vi "get.vi"(7 "save_to_file":path, 8 "error in (no error)":errorcluster, 10 "url":string, 11 "Client in":refnum<class "Client.lvclass">) -> (0 "error out":errorcluster, 2 "string_value":string, 3 "Client out":refnum<class "Client.lvclass">)   [LabVIEW 2020, in "reqwest.lvlib" / "Client.lvclass"]
uses:
  Client.lvclass
  Client.lvclass/Client.ctl
  lv_reqwest_64.dll
  reqwest.lvlib
  <userlib>/_OpenG.lib/file/file.llb/openg_file.lvlib
  <userlib>/_OpenG.lib/file/file.llb/Valid Path - Traditional__ogtk.vi
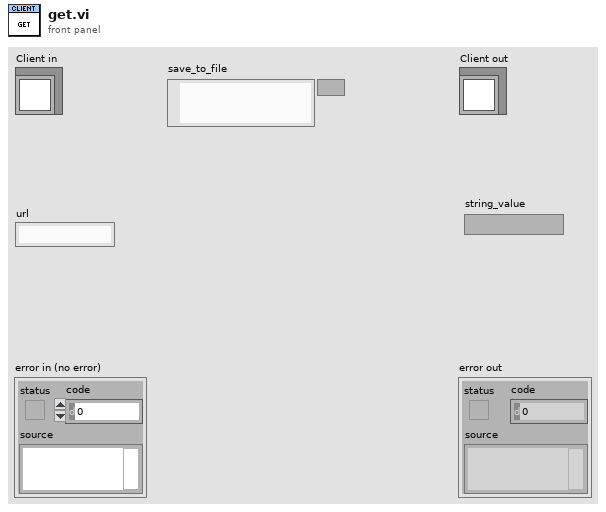
[diagram p1: front panel]
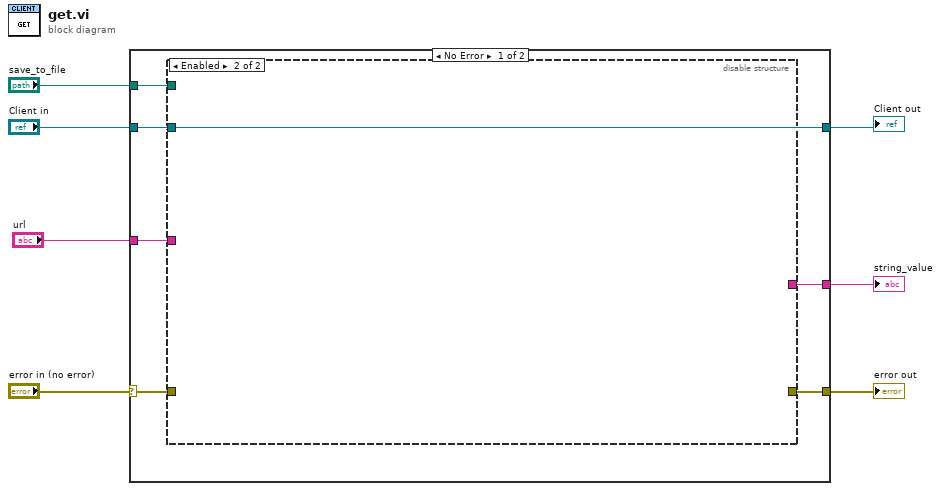
[diagram p0: block diagram]
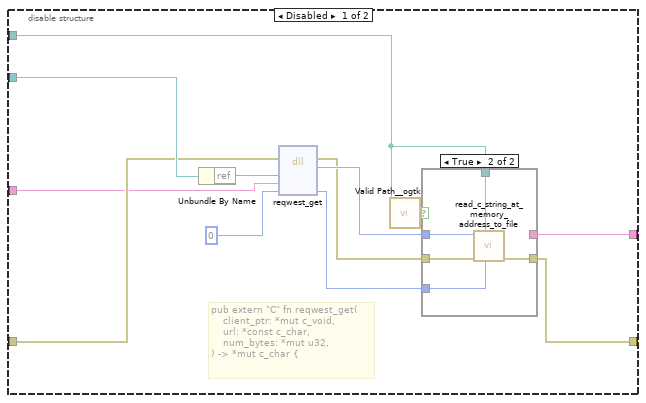
[diagram p2: hidden frame]
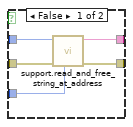
[diagram p3: hidden frame]
diagram:
  n1 = case shown="No Error" "error in (no error)" {
    selector: "error in (no error)" -> [w12 w36]
    tunnel: "Client in" -> [w13 w37]
    tunnel: [w9 _] -> w5
    tunnel: [w10 w36] -> w3
    tunnel: [w13 w37] -> w4
    tunnel: "url" -> [w11 _]
    tunnel: "save_to_file" -> [w8 _]
    frame No Error {
      n2 = disable-structure shown="Enabled" {
        disable-tunnel: w13 -> [w24 _]
        disable-tunnel: w12 -> [w23 _]
        disable-tunnel: w11 -> [w21 _]
        disable-tunnel: [w18 _] -> w10
        disable-tunnel: [w17 _] -> w9
        disable-tunnel: w8 -> [w14 _]
        frame Disabled {
          # "pub extern \"C\" fn reqwest_get(\n    client_ptr: *mut c_void,\n    url: *const c_char,\n    num_bytes: *mut u32,\n) -> *mut c_char {"
          n3 = Unbundle By Name(w24) -> ("ref"=w25:u64)
          n4 = dll-call lib="C:/Projects/reqwest-rs-labview/lv_src/lv_reqwest_64.dll" fn="reqwest_get"(error in=w23, "client_ref"=w25, "url"=w21, "num_bytes"=u32 0) -> (error out=w15:errorcluster, "string_ptr"=w16:u64, "num_bytes"=w19:u32)  [unwired: 4 in, 1 out]
          n5 = call-poly <userlib>:"Valid Path__ogtk.vi"("path"=w14) -> ("valid"=w20:bool)
          n6 = case shown="True" w20 {
            tunnel: w16 -> [w30 w33]
            tunnel: w15 -> [w29 w35]
            tunnel: [w28 _] -> w17
            tunnel: [w27 w34] -> w18
            tunnel: w19 -> [w26 w32]
            tunnel: w14 -> [_ w31]
            frame False {
              n7 = call "support.read_and_free_string_at_address.vi"("string_length"=w26, "error in (no error)"=w29, "string_ptr"=w30) -> ("error out"=w27:errorcluster, "string"=w28:string)  [unwired: 7 in]
            }
            frame True {
              n8 = call "read_c_string_at_memory_address_to_file.vi"("string_length"=w32, "File Path"=w31, "error in (no error)"=w35, "memory_address"=w33) -> ("error out"=w34:errorcluster)  [unwired: 6 in, 1 out]
            }
          }
        }
        frame Enabled {
        }
      }
    }
    frame Error {
    }
  }
  "error out" <- w3
  "string_value" <- w5
  "Client out" <- w4
